vi "get max string length in loop.vi"(11 "String":string) -> (3 "max length":i32)   [LabVIEW 2016, in "FPGA Resource Manager.lvlib"]
uses:
  FPGA Resource Manager.lvlib
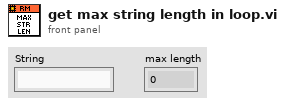
[diagram p1: front panel]
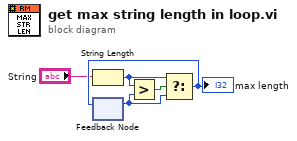
[diagram p0: block diagram]
diagram:
  n1 = String Length(string="String") -> (length=w4:i32)
  n2 = feedback #1() -> (w1:i32)  [unwired: 1 in]
  n3 = Greater?(x=w4, y=w1) -> (0:w3:bool)
  n4 = Select(t=w4, s=w3, f=w1) -> (s? t:f=w5:i32)
  "max length" <- w5
  n5 = feedback-in #1(w5) -> ()
